vi "GetOutputJSONPath.vi"(8 "error in (no error)":errorcluster, 11 "ConverterBase in":refnum<class "FileConverterBase.lvclass">) -> (0 "error out":errorcluster, 2 "Path":path, 3 "ConverterBase out":refnum<class "FileConverterBase.lvclass">)   [LabVIEW 2017, in "FileConverterBase.lvclass"]
uses:
  FileConverterBase.lvclass
  PathConfiguration.vi
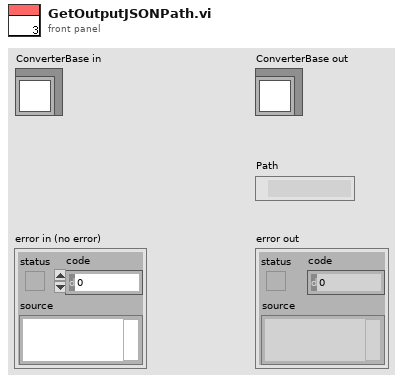
[diagram p1: front panel]
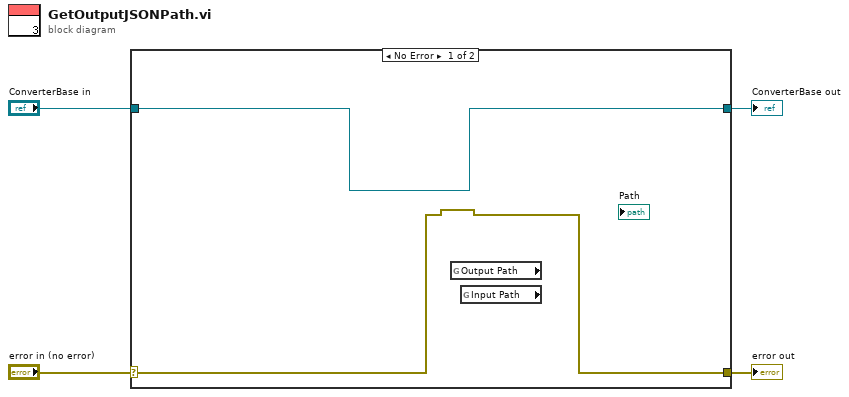
[diagram p0: block diagram]
diagram:
  n1 = case shown="No Error" "error in (no error)" {
    selector: "error in (no error)" -> [w5 w8]
    tunnel: [w5 w8] -> w3
    tunnel: [w6 w7] -> w1
    tunnel: "ConverterBase in" -> [w6 w7]
    frame No Error {
      n2 = global read "PathConfiguration.vi" "Output Path"() -> ()  [unwired: 1 out]
      n3 = global read "PathConfiguration.vi" "Input Path"() -> ()  [unwired: 1 out]
    }
    frame Error {
    }
  }
  "error out" <- w3
  "ConverterBase out" <- w1
